vi "List Buckets.vi"(8 "error in (no error)":errorcluster, 11 "AWS Credentials":T1) -> (0 "error out":errorcluster, 3 "Buckets":refnum<class "Bucket.lvclass">[](array[class]))   [LabVIEW 2015, in "NI_AWS_S3.lvlib" / "Bucket.lvclass"]
uses:
  Bucket.lvclass
  Core/HTTP Request/AWS Credentials.ctl
  Core/HTTP Request/Request Options.ctl
  Core/HTTP Request/Name Value Pair.ctl
  Core/HTTP Request/Region handling.ctl
  Core/HTTP Request/URL formatting.ctl
  Core/HTTP Request/HTTP Request.lvclass/HTTP Request.ctl
  Bucket.lvclass/Bucket.ctl
  Write Name.vi
  Core/HTTP Request/Write Credentials.vi
  Core/HTTP Request/Write Service.vi
  Core/HTTP Request/Write Verify Server.vi
  Core/HTTP Request/HTTP Request.lvclass
panel:
  out "Owner display name":string
  out "Owner ID":string
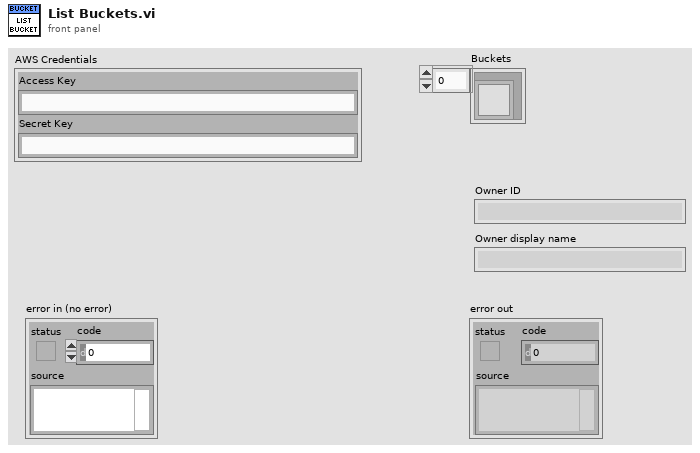
[diagram p1: front panel]
types:
  T1 = typedef "NI_AWS_Core.lvlib/HTTP Request.lvclass/AWS Credentials.ctl" = cluster{"Access Key":string, "Secret Key":string}
  T2 = typedef "NI_AWS_Core.lvlib/HTTP Request.lvclass/Region handling.ctl" = enum16{"use region everywhere", "use region (authentication only)", "use region (URL only)", "ignore region everwhere"}
  T3 = typedef "NI_AWS_Core.lvlib/HTTP Request.lvclass/Request Options.ctl" = cluster{"request headers":T4[], "request parameters":T4[], "request body":string, "region handling":T2, "URL formatting":T5}
  T4 = typedef "NI_AWS_Core.lvlib/HTTP Request.lvclass/Name Value Pair.ctl" = cluster{"name":string, "value":string}
  T5 = typedef "NI_AWS_Core.lvlib/HTTP Request.lvclass/URL formatting.ctl" = enum16{"region-", "region."}
  T6 = typedef "NI_AWS_Core.lvlib/HTTP Request.lvclass/Response.ctl" = cluster{"Headers":string, "Body":string}
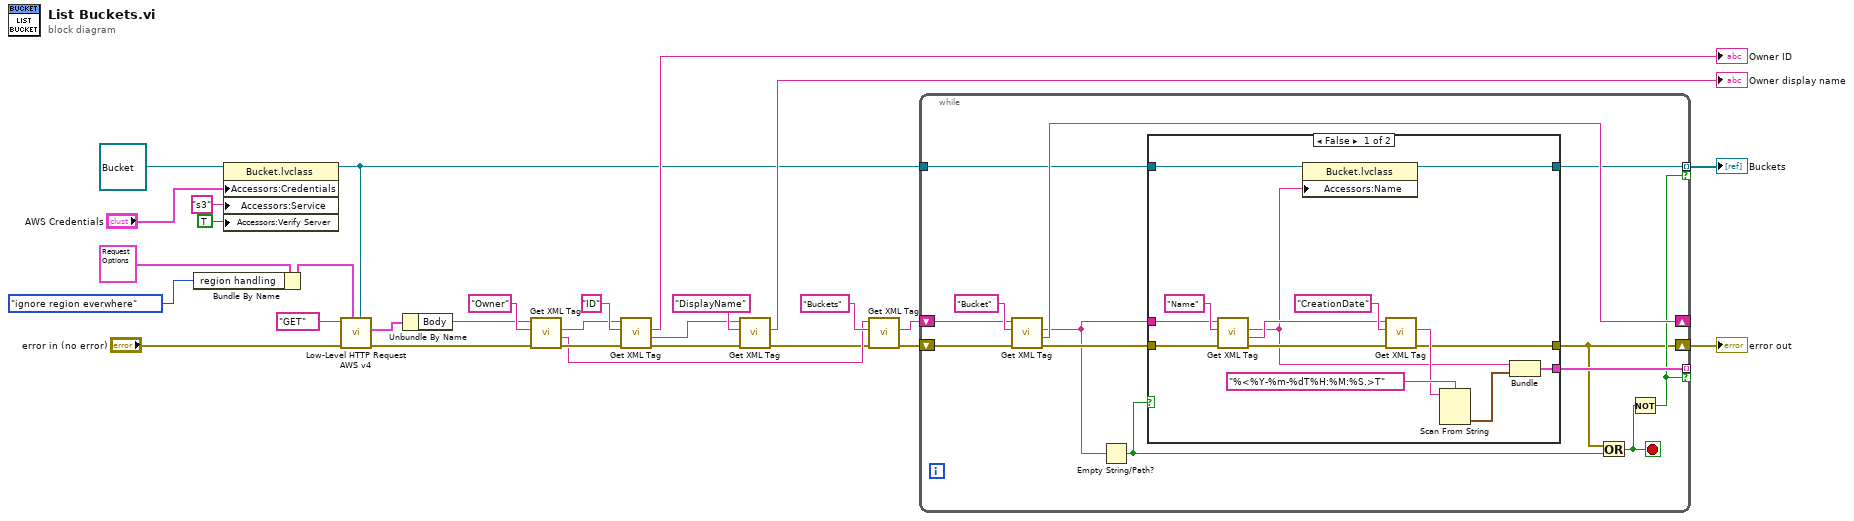
[diagram p0: block diagram]
diagram:
  n1 = Bundle By Name(cluster=T3 {"request headers"=[], "request parameters"=[], "request body"="", "region handling"=enum."use region everywhere", "URL formatting"=enum."region."} ("Request Options"), "region handling"=Region_handling."ignore region everwhere") -> (w2:T3)
  n2 = property class="Bucket.lvclass"(reference=refnum<class "Bucket.lvclass"> refnum ("NI_AWS_S3.lvlib:Bucket.lvclass"), "Accessors:Credentials"="AWS Credentials", "Accessors:Service"="s3" ("Service"), "Accessors:Verify Server"=TRUE ("Verify Server")) -> (reference out=w5:refnum<class "Bucket.lvclass">)  [unwired: 1 in, 1 out]
  n3 = call "Low-Level HTTP Request AWS v4.vi"("AWS Core"=w5, "Request Options"=w2, "error in (no error)"="error in (no error)", "HTTP-Verb"="GET") -> ("error out"=w6:errorcluster, "Response"=w29:T6)  [unwired: 5 in, 1 out]
  n4 = Unbundle By Name(w29) -> ("Body"=w13:string)
  n5 = call "Get XML Tag.vi"("error in (no error)"=w6, "Tag name"="Owner", "XML String in"=w13) -> ("error out"=w16:errorcluster, "Remaining string"=w12:string, "Tag value"=w14:string)  [unwired: 4 in, 2 out]
  n6 = call "Get XML Tag.vi"("error in (no error)"=w16, "Tag name"="ID", "XML String in"=w14) -> ("error out"=w15:errorcluster, "Remaining string"=w11:string, "Tag value"=→"Owner ID":string)  [unwired: 4 in, 2 out]
  n7 = call "Get XML Tag.vi"("error in (no error)"=w15, "Tag name"="DisplayName", "XML String in"=w11) -> ("error out"=w7:errorcluster, "Tag value"=→"Owner display name":string)  [unwired: 4 in, 3 out]
  n8 = call "Get XML Tag.vi"("error in (no error)"=w7, "Tag name"="Buckets", "XML String in"=w12) -> ("error out"=w21:errorcluster, "Tag value"=w10:string)  [unwired: 4 in, 3 out]
  n9 = while {
    shift-right: [w38] -> _
    shift-left: w10 -> [w41]
    shift-right: [w33] -> w17
    shift-left: w21 -> [w40]
    tunnel: [w37] -> _ mode=indexing if=w34
    tunnel: w5 -> [w35]
    tunnel: [w30] -> w4 mode=indexing if=w34
    stop <- w31 stop-if-true
    n10 = call "Get XML Tag.vi"("error in (no error)"=w40, "Tag name"="Bucket", "XML String in"=w41) -> ("error out"=w39:errorcluster, "Remaining string"=w38:string, "Tag value"=w36:string)  [unwired: 4 in, 2 out]
    n11 = Empty String/Path?(string/path=w36) -> (empty?=w32:bool)
    n12 = case shown="False" w32 {
      tunnel: w39 -> [w51 w57]
      tunnel: [w44 w57] -> w33
      tunnel: [w49 _] -> w37
      tunnel: w36 -> [w48 _]
      tunnel: w35 -> [w47 _]
      tunnel: [w43 _] -> w30
      frame False {
        n13 = call "Get XML Tag.vi"("error in (no error)"=w51, "Tag name"="Name", "XML String in"=w48) -> ("error out"=w52:errorcluster, "Remaining string"=w46:string, "Tag value"=w45:string)  [unwired: 4 in, 2 out]
        n14 = property class="Bucket.lvclass"(reference=w47, "Accessors:Name"=w45) -> (reference out=w43:refnum<class "Bucket.lvclass">)  [unwired: 1 in, 1 out]
        n15 = call "Get XML Tag.vi"("error in (no error)"=w52, "Tag name"="CreationDate", "XML String in"=w46) -> ("error out"=w44:errorcluster, "Tag value"=w53:string)  [unwired: 4 in, 3 out]
        n16 = Scan From String(format string="%<%Y-%m-%dT%H:%M:%S.>T", input string=w53) -> (output 1=w50:timestamp)  [unwired: 3 in, 3 out]
        n17 = Bundle("Tag value"=w45, w50) -> (w49:cluster{"Tag value":string, timestamp})  [unwired: 1 in]
      }
      frame True {
      }
    }
    n18 = Or(x=w33, y=w32) -> (x .or. y?=w31:bool)
    n19 = Not(x=w31) -> (.not. x?=w34:bool)
  }
  "error out" <- w17
  "Buckets" <- w4
